vi "SAOMM-Astrometry.vi"(0 "Binning":u16(ring) items=["1 x 1"=1, "2 x 2"=2, "4 x 4"=4, "5 x 5"=5], 1 "PIXSCALE":cluster{"pixscale2":dbl, "pixscale1":dbl}, 2 "NAXIS":cluster{"naxis2":u16, "naxis1":u16}, 11 "Rotation":dbl format="%.1f", 12 "RAsonde":dbl format="%<%H:%M:%S%1u>t", 13 "DECsonde":dbl format="%<%H:%M:%S>t") -> (8 "GuideAstrom":T1 {"CRVAL" format="%.6g"; "CD" format="%_7g"})   [LabVIEW 2019]
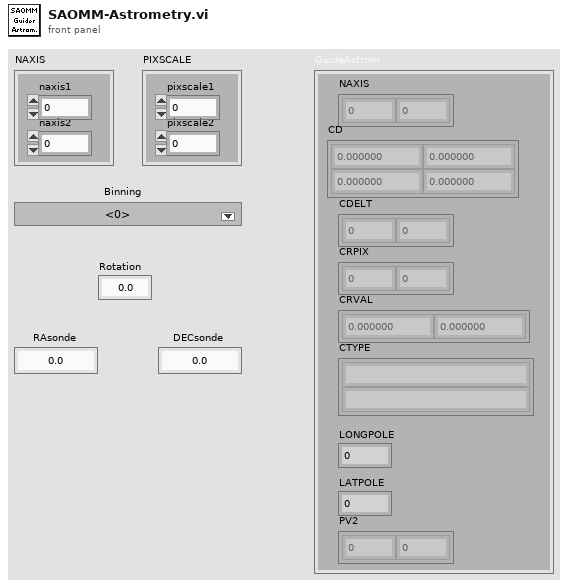
[diagram p1: front panel]
types:
  T1 = cluster{"NAXIS":dbl[], "CD":dbl[][], "CDELT":dbl[], "CRPIX":dbl[], "CTYPE":string[], "CRVAL":dbl[], "LONGPOLE":dbl, "LATPOLE":dbl, "PV2":dbl[]}
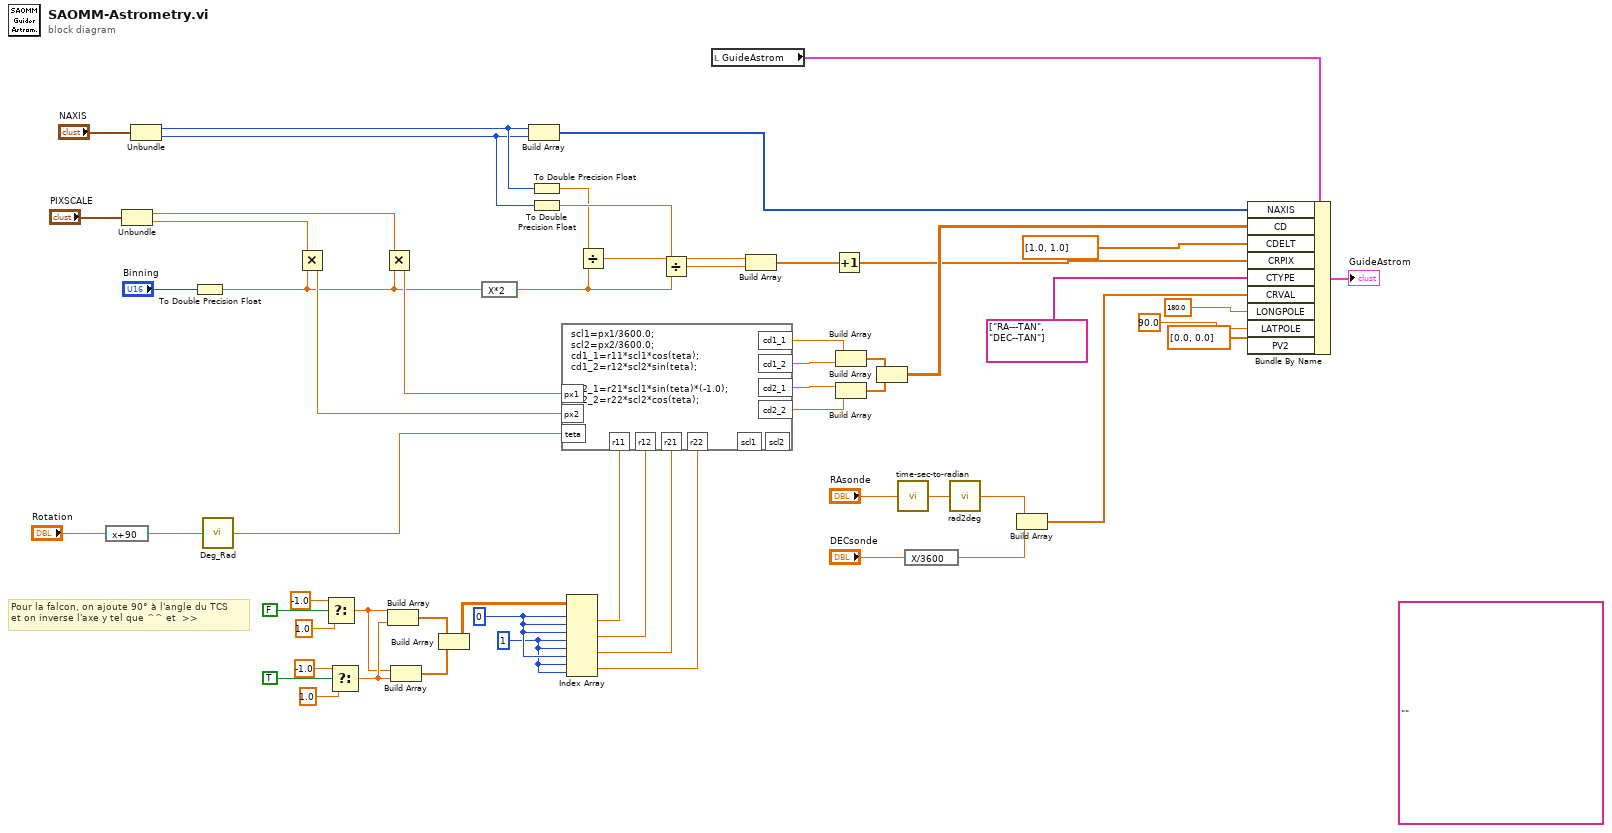
[diagram p0: block diagram]
diagram:
  (unwired) ""
  w43 = 1 ("disabled index (col)")
  w44 = 0 ("index (row)")
  # "Pour la falcon, on ajoute 90° à l'angle du TCS\net on inverse l'axe y tel que ^^ et  >>"
  n1 = expression code="x+90"("Rotation") -> (w3:dbl)
  n2 = Unbundle("PIXSCALE") -> ("pixscale2"=w22:dbl, "pixscale1"=w37:dbl)
  n3 = Unbundle("NAXIS") -> ("naxis2"=w8:u16, "naxis1"=w7:u16)
  n4 = To Double Precision Float(number="Binning") -> (double precision float=w23:dbl)
  n5 = call "Deg_Rad.vi"("Angle"=w3) -> ("RadRot"=w34:dbl)
  n6 = Multiply(x=w37, y=w23) -> (x*y=w35:dbl)
  n7 = Select(t=-1.0, s=FALSE ("Inv Y"), f=1.0 ("t")) -> (s? t:f=w48:dbl)
  n8 = Select(t=-1.0, s=TRUE ("Inv Y"), f=1.0 ("t")) -> (s? t:f=w51:dbl)
  n9 = Multiply(x=w22, y=w23) -> (x*y=w36:dbl)
  n10 = Build Array(w48, w51) -> (w53:dbl[])
  n11 = Build Array(w48, w51) -> (w52:dbl[])
  n12 = Build Array(w53, w52) -> (w45:dbl[][])
  n13 = expression code="X*2"(w23) -> (w21:dbl)
  n14 = Build Array(w8, w7) -> (w54:u16[])
  n15 = To Double Precision Float(number=w8) -> (double precision float=w5:dbl)
  n16 = To Double Precision Float(number=w7) -> (double precision float=w6:dbl)
  n17 = Index Array(array=w45, index (row) #1=w44, index (col) #1=w44, index (row) #2=w44, index (col) #2=w43, index (row) #3=w43, index (col) #3=w44, index (row) #4=w43, index (col) #4=w43) -> (element #1=w42:dbl, element #2=w41:dbl, element #3=w40:dbl, element #4=w39:dbl)
  n18 = formula code="scl1=px1/3600.0;\nscl2=px2/3600.0;\ncd1_1=r11*scl1*cos(teta);\ncd1_2=r12*scl2*sin(teta);\n\ncd2_1=r21*scl1*sin(teta)*(-1.0);\ncd2_2=r22*scl2*cos(teta);"("teta"=w34, "px1"=w36, "r11"=w42, "r12"=w41, "r21"=w40, "r22"=w39, "px2"=w35) -> ("cd1_1"=w31:dbl, "cd1_2"=w30:dbl, "cd2_1"=w29:dbl, "cd2_2"=w28:dbl)  [unwired: 2 out]
  n19 = Divide(x=w5, y=w21) -> (x/y=w20:dbl)
  n20 = Divide(x=w6, y=w21) -> (x/y=w19:dbl)
  n21 = local read "GuideAstrom"() -> (w58:T1)
  n22 = Build Array(w20, w19) -> (w18:dbl[])
  n23 = Increment(x=w18) -> (x+1=w17:dbl[])
  n24 = Build Array(w31, w30) -> (w32:dbl[])
  n25 = Build Array(w29, w28) -> (w33:dbl[])
  n26 = Build Array(w32, w33) -> (w27:dbl[][])
  n27 = call "time-sec-to-radian.vi"("Numeric"="RAsonde") -> ("radians"=w16:dbl)
  n28 = expression code="X/3600"("DECsonde") -> (w12:dbl)
  n29 = call "rad2deg.vi"("rad"=w16) -> ("deg"=w14:dbl)
  n30 = Build Array(w14, w12) -> (w25:dbl[])
  n31 = Bundle By Name(cluster=w58, "NAXIS"=w54, "CD"=w27, "CDELT"=dbl[] [1.0, 1.0], "CRPIX"=w17, "CTYPE"=string[] ["RA---TAN", "DEC--TAN"], "CRVAL"=w25, "LONGPOLE"=180.0, "LATPOLE"=90.0, "PV2"=dbl[] [0.0, 0.0]) -> (→"GuideAstrom":T1)
